vi "Day 9.vi"() -> ()   [LabVIEW 2021]
uses:
  e82450e5-71a3-46d6-8b92-650601a06453.vi
  <vilib>/Utility/file.llb/Read Delimited Spreadsheet (string).vi
  <vilib>/Comparison/Less/Less Functor/Less Functor.lvclass
panel:
  out "Data":i32[][](array[numeric])
  out "Intensity Graph":i32[][](graph)
  out "Solution":i32
  in  "Input File":enum32{"example input", "input"}(radio)
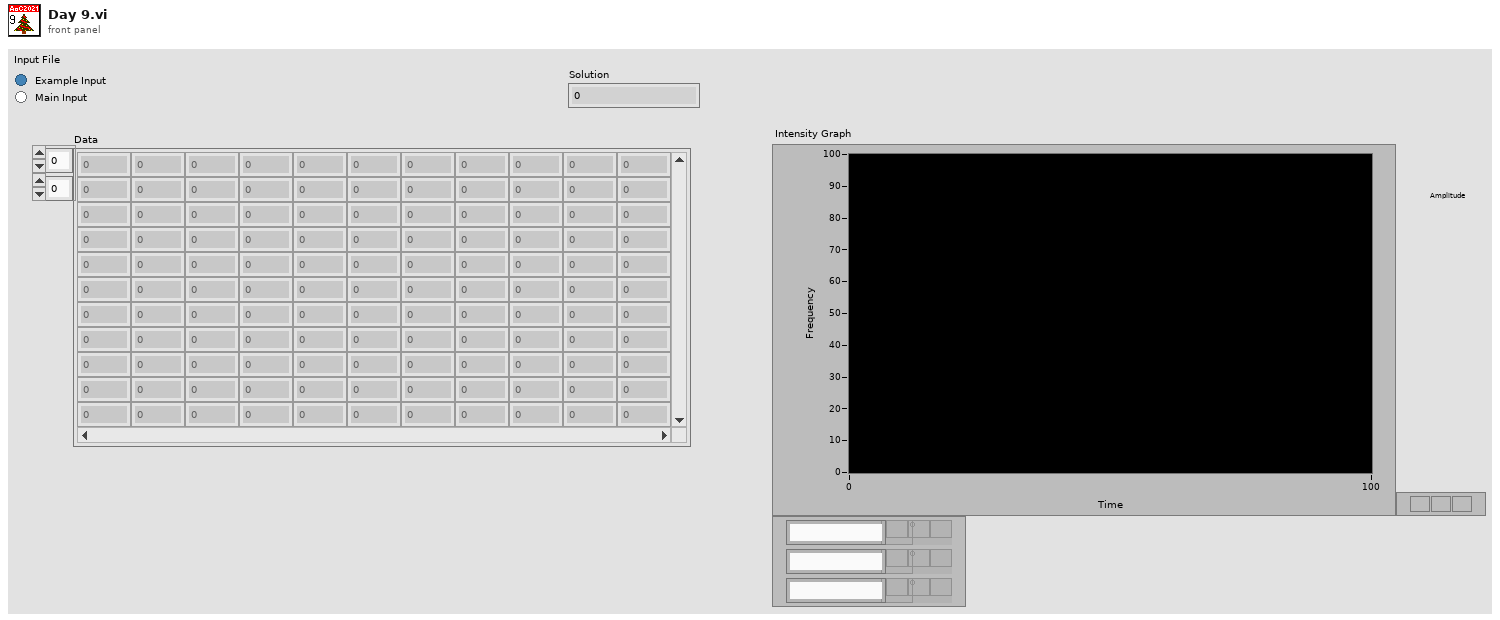
[diagram p1: front panel]
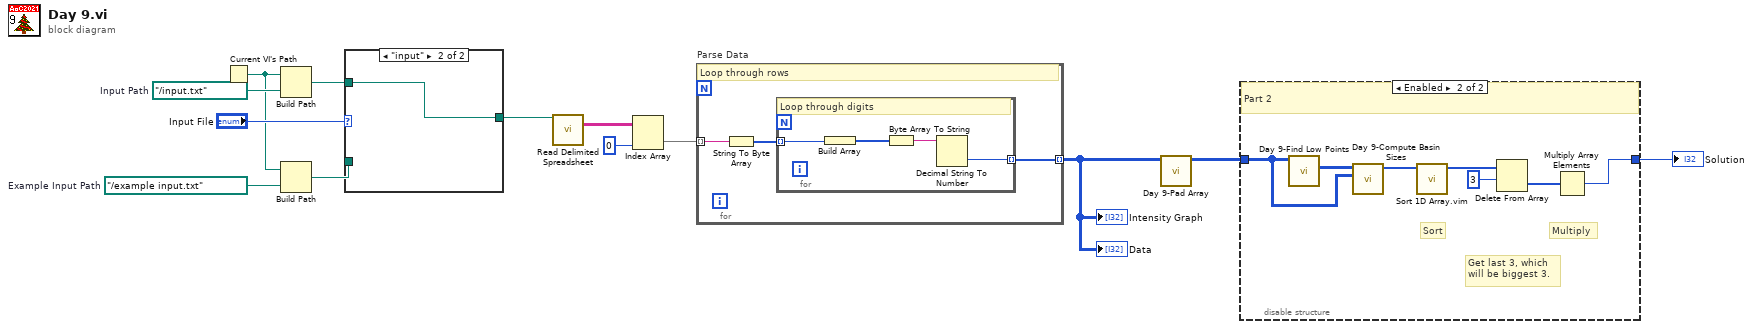
[diagram p0: block diagram]
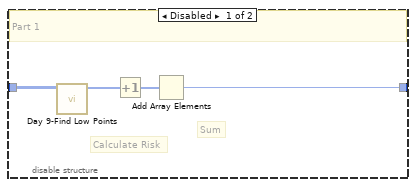
[diagram p3: hidden frame]
diagram:
  w12 = path "../example input.txt"  # Example Input Path
  w13 = path "../input.txt"  # Input Path
  n1 = Current VI's Path() -> (path=w7:path)
  n2 = Build Path(base path=w7, name or relative path=w13) -> (appended path=w10:path)
  n3 = Build Path(base path=w7, name or relative path=w12) -> (appended path=w9:path)
  n4 = case shown="\"input\"" "Input File" {
    tunnel: w10 -> [_ w15]
    tunnel: w9 -> [w14 _]
    tunnel: [w14 w15] -> w8
    frame "example input" {
    }
    frame "input" {
    }
  }
  n5 = call-poly <vilib>:"Read Delimited Spreadsheet.vi"("file path (dialog if empty)"=w8) -> ("all rows"=w6:string[][])  [unwired: 9 in, 5 out]
  n6 = Index Array(array=w6, index (col)=0 ("disabled index (col)")) -> (element=w4:string[])  [unwired: 1 in]
  n7 = for "Parse Data" {
    tunnel: w4 -> [w18] mode=indexing
    tunnel: [w16] -> w2 mode=indexing
    # "Loop through rows"
    n8 = String To Byte Array(string=w18) -> (unsigned byte array=w17:u8[])
    n9 = for {
      tunnel: w17 -> [w22] mode=indexing
      tunnel: [w19] -> w16 mode=indexing
      # "Loop through digits"
      n10 = Build Array(w22) -> (w21:u8[])
      n11 = Byte Array To String(unsigned byte array=w21) -> (string=w20:string)
      n12 = Decimal String To Number(string=w20) -> (number=w19:i32)  [unwired: 2 in, 1 out]
    }
  }
  "Intensity Graph" <- w2
  "Data" <- w2
  n13 = call "Day 9-Pad Array.vi"("Array in"=w2) -> ("Array out"=w1:i32[][])  [unwired: 10 in]
  n14 = disable-structure shown="Enabled" {
    disable-tunnel: [w26 w29] -> w3
    disable-tunnel: w1 -> [w24 w27]
    frame Disabled {
      # "Sum"
      # "Calculate Risk"
      # "Part 1"
      n15 = call "Day 9-Find Low Points.vi"("Array in"=w24) -> ("Low Point Values"=w23:i32[])  [unwired: 9 in, 1 out]
      n16 = Increment(x=w23) -> (x+1=w25:i32[])
      n17 = Add Array Elements(numeric array=w25) -> (sum=w26:i32)
    }
    frame Enabled {
      # "Multiply"
      # "Get last 3, which will be biggest 3."
      # "Sort"
      # "Part 2"
      n18 = call "Day 9-Find Low Points.vi"("Array in"=w27) -> ("Low Point Coordinates"=w28:i32[][])  [unwired: 9 in, 1 out]
      n19 = call "Day 9-Compute Basin Sizes.vi"("Padded Data Array in"=w27, "Low Point Coordinates"=w28) -> ("All Basin Sizes"=w33:i32[])  [unwired: 9 in]
      n20 = call "Sort 1D Array.vim"("unsorted array"=w33) -> ("sorted array"=w32:i32[])  [unwired: 10 in]
      n21 = Delete From Array(array=w32, length=3) -> (deleted portion=w30:i32[])  [unwired: 1 in, 1 out]
      n22 = Multiply Array Elements(1:w30) -> (0:w29:i32)
    }
  }
  "Solution" <- w3
